vi "624 Ball Detection.vi"(8 "Color Components Refnum":refnum<vi>, 9 "Image In":T1, 10 "Score Cutoff":dbl(slide)=70.58823529411765 scale=0.0..100.0, 11 "Image Ctl Refnum":refnum<vi>) -> (0 "Diameter":sgl, 1 "Y":sgl, 2 "Ball Found?":bool, 3 "X":sgl, 4 "Image":T1(plugin-control), 5 "Initial Mask":T1(plugin-control))   [LabVIEW 2013]
uses:
  <vilib>/vision/Image Controls.llb/IMAQ Image.ctl
panel:
  in  "Std Devs":cluster{"Hue":dbl, "Sat":dbl, "Val":dbl}={"Hue"=4.0, "Sat"=6.0, "Val"=4.0}
  in  "Targets":i32=3
  in  "Area Size Limit %":dbl=0.4 format="%#_13g"
  in  "Instructions:":string="Use the tab immediately below to choose the image source. Update the camera settings or the image directory so that you have images or video to test with.\n\nCalibration:\nYou can update Color Component ranges directly, or by clicking and drawing a line across the upper third of a ball within the image -- example shown below-right.\n\nUse Debugging tab to view intermediate results. Adjust Std Dev multipliers and line to achieve the desired HSV upper and lower threshold limits.\n\nArea Size LImit is used to ignore objects too small or balls too far away to care about.\n\nTargets identifies how many of the top scores to return.\n\nThe Details tab contains center, radius, and score details of each object."
  out "Color Components":T2={"Hue"={243.23333311080933, 20.233333110809326}, "Sat"={125.60287475585938, 242.93045043945312}, "Val"={83.88507843017578, 225.38158416748047}} {"Val" scale=0.0..255.0; "Sat" scale=0.0..255.0; "Hue" scale=0.0..255.0 scale format="%#_3g"}
  in  "Tabbed Info":enum32{"Debugging", "Details"}(tab)
  in  "Annotations":enum16{"None", "Good", "All"}(ring)=enum."Good"
  out "Fitted Mask":T1(plugin-control)
  out "Ranked Objects":T3(array[cluster]) {"Score" format="%#.1g"}
  # "Ranking Colors:\n1. green\n2. cyan\n3. magenta\n4. orange"
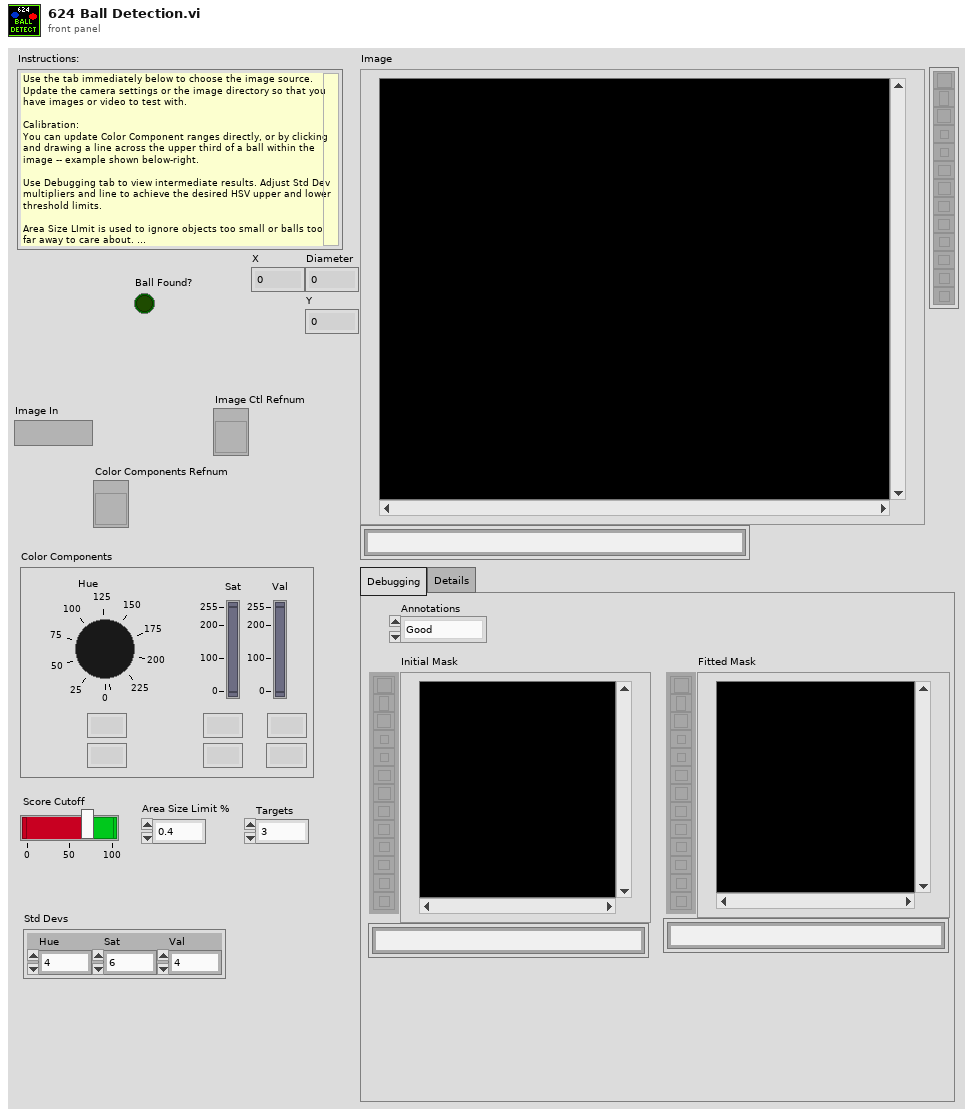
[diagram p1: front panel]
types:
  T1 = typedef "IMAQ Image.ctl" = refnum<image>
  T2 = cluster{"Hue":cluster{dbl, dbl}, "Sat":cluster{dbl, dbl}, "Val":cluster{dbl, dbl}}
  T3 = cluster{"Score":sgl, "Fitted Circle":cluster{"Center":cluster{"X":sgl, "Y":sgl}, "Radius":dbl, "Circle Rect":cluster{"L":sgl, "T":sgl, "R":sgl, "B":sgl}, "Roundness":dbl, "SNR (dB)":dbl}, "Search Rect":cluster{"L":sgl, "T":sgl, "R":sgl, "B":sgl}, "Details":cluster{"Edge":sgl, "Area":sgl, "Circ":sgl, "Diam":sgl}}[]
  T4 = cluster{"Circle Found":bool, "Fitted Circle":cluster{"Center":cluster{"X":sgl, "Y":sgl}, "Radius":dbl, "Center":cluster{"X":sgl, "Y":sgl}, "Radius":dbl, "Roundness":dbl, "Strength":dbl, "SNR (dB)":dbl}, "Array":dbl[], "Sorted Data":dbl[][]}[]
  T5 = cluster{cluster{dbl, dbl}, cluster{dbl, dbl}, cluster{dbl, dbl}}
  T6 = cluster{"Score":dbl, "Fitted Circle":cluster{"Center (Pixels)":cluster{"X":sgl, "Y":sgl}, "Radius (Pixels)":dbl, "Circle Rect":cluster{"Left":sgl, "Top":sgl, "Right":sgl, "Bottom":sgl}, "Roundness (RW)":dbl, "Average SNR (dB)":dbl}, "Search Rect":cluster{"Left":sgl, "Top":sgl, "Right":sgl, "Bottom":sgl}, "Details":cluster{"Edges":sgl, "Circ/Rect":sgl, "Diam/Diam":sgl, "Circularity":sgl}}[]
  T7 = cluster{"Score":dbl, "Fitted Circle":cluster{"Center (Pixels)":cluster{"X":sgl, "Y":sgl}, "Radius (Pixels)":dbl, "Circle Rect":cluster{"Left":sgl, "Top":sgl, "Right":sgl, "Bottom":sgl}, "Roundness (RW)":dbl, "Average SNR (dB)":dbl}, "Search Rect":cluster{"Left":sgl, "Top":sgl, "Right":sgl, "Bottom":sgl}, "Details":cluster{"Edges":sgl, "Circ/Rect":sgl, "Diam/Diam":sgl, "Circularity":sgl}}
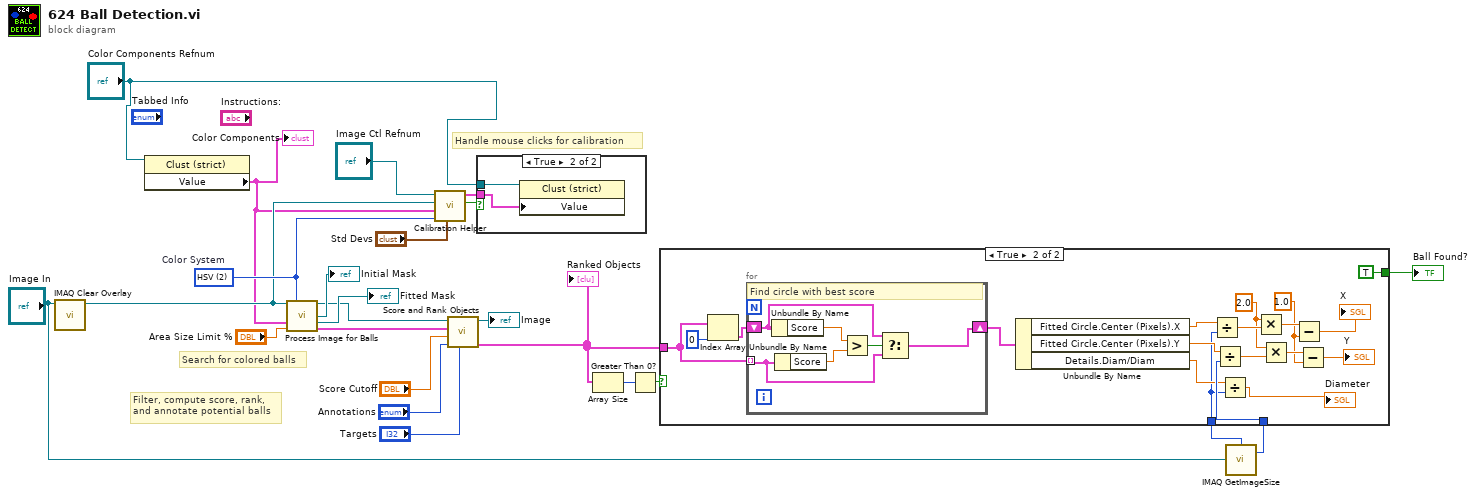
[diagram p0: block diagram]
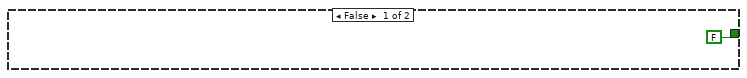
[diagram p2: hidden frame]
diagram:
  w21 = u16 2 items=["RGB", "HSL", "HSV", "HSI"]  # Color System
  # "Handle mouse clicks for calibration"
  # "Search for colored balls"
  # "Filter, compute score, rank,\nand annotate potential balls"
  n1 = call "IMAQ Clear Overlay"("Image"="Image In") -> ("Image Out"=w14:T1)  [unwired: 9 in, 1 out]
  n2 = property class="Clust (strict)"(reference="Color Components Refnum") -> ("Value"=w1:T2)  [unwired: 1 in, 2 out]
  "Color Components" <- w1
  n3 = call "Process Image for Balls.vi"("Src Image"=w14, "Color Mode 2"=w21, "Color"=w1, "Area Cutoff %"="Area Size Limit %") -> ("Src Image Out"=w16:T1, "First Threshold"=→"Initial Mask":T1, "Fitted"=→"Fitted Mask":T1, "Potential"=w17:T4)  [unwired: 8 in]
  n4 = call "Calibration Helper.vi"("Std Devs"="Std Devs", "Color Mode"=w21, "Color Components"=w1, "Image"=w14, "Image Ctl Refnum"="Image Ctl Refnum") -> ("Changed"=w24:bool, "output color"=w22:T5)  [unwired: 5 in]
  n5 = call "Score and Rank Objects.vi"("Targets"="Targets", "Annotations"="Annotations", "Score Limit"="Score Cutoff", "Object Info"=w17, "Image in"=w16) -> ("Object Info"=w6:T6, "Annotated Image"=→"Image":T1)  [unwired: 5 in]
  "Ranked Objects" <- w6
  n6 = case shown="True" w24 {
    tunnel: w22 -> [_ w26]
    tunnel: "Color Components Refnum" -> [_ w25]
    frame False {
    }
    frame True {
      n7 = property class="Clust (strict)"(reference=w25, "Value"=w26) -> ()  [unwired: 1 in, 2 out]
    }
  }
  n8 = Array Size(array=w6) -> (size(s)=w5:i32)
  n9 = Greater Than 0?(x=w5) -> (x > 0?=w4:bool)
  n10 = call "IMAQ GetImageSize"("Image"="Image In") -> ("Y Resolution"=w8:i32, "X Resolution"=w7:i32)  [unwired: 3 in, 1 out]
  n11 = case shown="True" w4 {
    tunnel: w8 -> [_ w40]
    tunnel: w7 -> [_ w33]
    tunnel: w6 -> [_ w29]
    tunnel: [FALSE TRUE] -> w3
    frame False {
    }
    frame True {
      w36 = sgl 1.0 ("y")
      w39 = sgl 2.0 ("x")
      n12 = Index Array(array=w29, index=0) -> (element=w45:T7)
      n13 = for {
        tunnel: w29 -> [w48] mode=indexing
        shift-right: [w47] -> w44
        shift-left: w45 -> [w50]
        # "Find circle with best score"
        n14 = Unbundle By Name(w50) -> ("Score"=w51:dbl)
        n15 = Unbundle By Name(w48) -> ("Score"=w49:dbl)
        n16 = Greater?(x=w51, y=w49) -> (0:w52:bool)
        n17 = Select(t=w50, s=w52, f=w48) -> (s? t:f=w47:T7)
      }
      n18 = Unbundle By Name(w44) -> ("Fitted Circle.Center (Pixels).X"=w43:sgl, "Fitted Circle.Center (Pixels).Y"=w41:sgl, "Details.Diam/Diam"=w34:sgl)
      n19 = Divide(x=w43, y=w33) -> (x/y=w42:sgl)
      n20 = Divide(x=w41, y=w40) -> (x/y=w35:sgl)
      n21 = Divide(x=w34, y=w33) -> (x/y=→"Diameter":sgl)
      n22 = Multiply(x=w39, y=w42) -> (x*y=w38:sgl)
      n23 = Multiply(x=w39, y=w35) -> (x*y=w37:sgl)
      n24 = Subtract(x=w38, y=w36) -> (x-y=→"X":sgl)
      n25 = Subtract(x=w37, y=w36) -> (x-y=→"Y":sgl)
    }
  }
  "Ball Found?" <- w3
